vi "BatteryWarningTest_3.6V.vi"(8 "error in":errorcluster) -> (0 "error in (no error)":errorcluster, 1 "Pass/Fail":bool, 4 "Limit2":u8[](array[numeric]) format="%x", 5 "Limit1":u8[](array[numeric]) format="%x")   [LabVIEW 2009]
uses:
  Global/Global 1.vi
  <vilib>/Instr/_visa.llb/VISA Configure Serial Port (Instr).vi
panel:
  # "30"
  # "0A"
  # "30"
  # "0A"
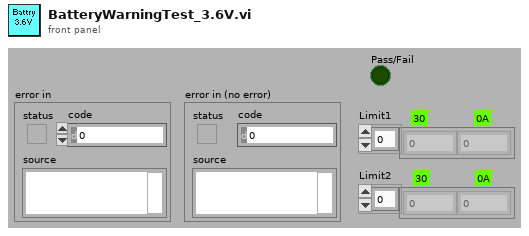
[diagram p1: front panel]
types:
  T1 = cluster{"VHEATFUSENOLOADMIN":string, "VHEATFUSELOADMAX":string, "VOVERRIDEDIODEMIN":string, "TDIFFMAX":string, "MEASFREQMAX":string, "MEASFREQMIN":string, "VOVER":string, "VMIDDLE":string, "VUNDER":string, "VNORESET":string, "VRESET":string, "WAITPING":string, "LRFID":string, "RFIDUID":string, "EXTEESIZE":string, "LCUTYPE":string, "LCUSUBTYPE":string, "TEVN":string, "BOOTVER":string, "APPVER":string, "ISLEEPMAX":string, "TSLEEP":string, "APPWAIT":string, "DBWAIT":string}
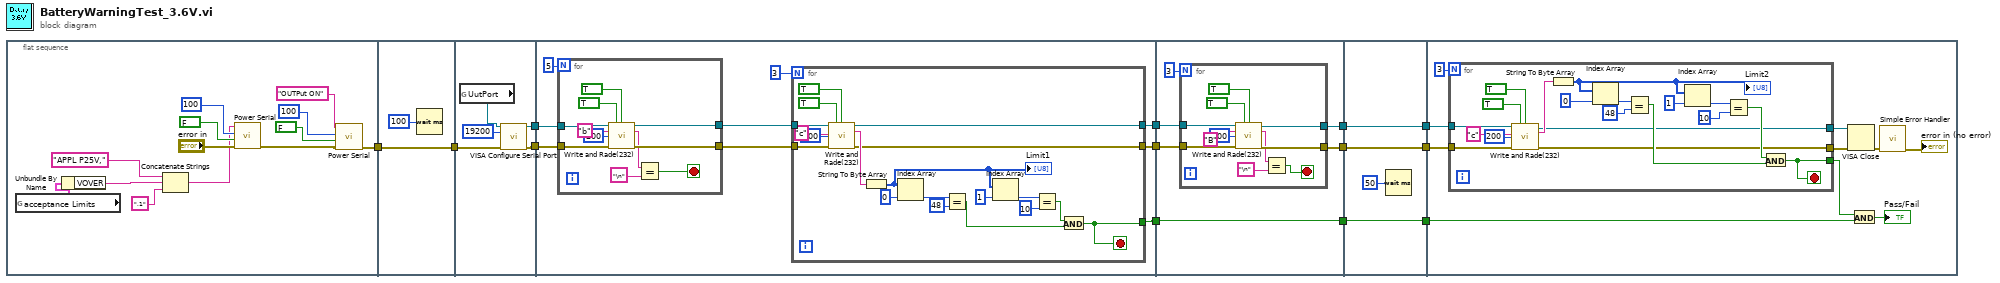
[diagram p0: block diagram]
diagram:
  n1 = flat-sequence {
    tunnel: [w19] -> w2
    tunnel: w2 -> [w28]
    tunnel: [w28] -> w1
    tunnel: [w33] -> w5
    tunnel: [w32] -> w4
    tunnel: w1 -> [w30]
    tunnel: [w42] -> w11
    tunnel: [w41] -> w6
    tunnel: [w38] -> w3
    tunnel: w4 -> [w35]
    tunnel: w5 -> [w36]
    tunnel: [w78] -> w12
    tunnel: w11 -> [w78]
    tunnel: [w77] -> w10
    tunnel: [w76] -> w8
    tunnel: w6 -> [w75]
    tunnel: w3 -> [w74]
    tunnel: [w92] -> w13
    tunnel: w12 -> [w92]
    tunnel: w10 -> [w91]
    tunnel: [w91] -> w9
    tunnel: w8 -> [w90]
    tunnel: [w90] -> w7
    tunnel: w13 -> [w102]
    tunnel: w9 -> [w100]
    tunnel: w7 -> [w99]
    frame #0 {
      n2 = global read "Global 1.vi" "acceptance Limits"() -> (w18:T1)
      n3 = Unbundle By Name(w18) -> ("VOVER"=w17:string)
      n4 = Concatenate Strings("APPL P25V," ("In"), w17, ",1" ("string")) -> (w14:string)
      n5 = call "Power Serial.vi"("error in (no error)"="error in", "Rd?"=FALSE, "Delay"=100, "IN"=w14) -> ("error out"=w23:errorcluster)  [unwired: 1 in, 6 out]
      n6 = call "Power Serial.vi"("error in (no error)"=w23, "Rd?"=FALSE, "Delay"=100, "IN"="OUTPut ON" ("In")) -> ("error out"=w19:errorcluster)  [unwired: 1 in, 6 out]
    }
    frame #1 {
      n7 = Wait (ms)(milliseconds to wait=u32 100) -> ()  [unwired: 1 out]
    }
    frame #2 {
      n8 = global read "Global 1.vi" "UutPort"() -> (w29:refnum<visa-resource-name>)
      n9 = call-poly "VISA Configure Serial Port"("VISA resource name"=w29, "baud rate (9600)"=u32 19200, "error in (no error)"=w30) -> ("VISA resource name out"=w32:refnum<visa-resource-name>, "error out"=w33:errorcluster)  [unwired: 3 in, 8 out]
    }
    frame #3 {
      n10 = for {
        N: 5 -> [_]
        tunnel: [w50] -> w40
        tunnel: w36 -> [w49]
        tunnel: w35 -> [w48]
        tunnel: [w47] -> w39
        stop <- w44 stop-if-true
        n11 = call "Write and Rade(232).vi"("VISA resource name in"=w48, "write"=TRUE, "read"=TRUE, "string to write"="b", "ms delay"=u32 200, "error in"=w49) -> ("VISA resource name out"=w50:refnum<visa-resource-name>, "read string"=w46:string, "error out"=w47:errorcluster)  [unwired: 2 in, 5 out]
        n12 = Equal?(x=w46, y="\n") -> (x = y?=w44:bool)
      }
      n13 = for {
        N: 3 -> [_]
        tunnel: [w55] -> w42
        tunnel: [w59] -> w41
        tunnel: w40 -> [w58]
        tunnel: w39 -> [w57]
        tunnel: [w56] -> w38
        stop <- w55 stop-if-true
        n14 = call "Write and Rade(232).vi"("VISA resource name in"=w58, "write"=TRUE, "read"=TRUE, "string to write"="c", "ms delay"=u32 200, "error in"=w57) -> ("VISA resource name out"=w59:refnum<visa-resource-name>, "read string"=w61:string, "error out"=w56:errorcluster)  [unwired: 2 in, 5 out]
        n15 = String To Byte Array(string=w61) -> (unsigned byte array=w67:u8[])
        "Limit1" <- w67
        n16 = Index Array(array=w67, index=0) -> (element=w65:u8)
        n17 = Equal?(x=w65, y=u8 48) -> (x = y?=w72:bool)
        n18 = Index Array(array=w67, index=1) -> (element=w69:u8)
        n19 = Equal?(x=w69, y=u8 10) -> (x = y?=w71:bool)
        n20 = And(x=w71, y=w72) -> (x .and. y?=w55:bool)
      }
    }
    frame #4 {
      n21 = for {
        N: 3 -> [_]
        tunnel: [w86] -> w77
        tunnel: [w85] -> w76
        tunnel: w75 -> [w84]
        tunnel: w74 -> [w83]
        stop <- w80 stop-if-true
        n22 = call "Write and Rade(232).vi"("VISA resource name in"=w84, "write"=TRUE, "read"=TRUE, "string to write"="B", "ms delay"=u32 200, "error in"=w83) -> ("VISA resource name out"=w85:refnum<visa-resource-name>, "read string"=w82:string, "error out"=w86:errorcluster)  [unwired: 2 in, 5 out]
        n23 = Equal?(x=w82, y="\n") -> (x = y?=w80:bool)
      }
    }
    frame #5 {
      n24 = Wait (ms)(milliseconds to wait=u32 50) -> ()  [unwired: 1 out]
    }
    frame #6 {
      n25 = for {
        N: 3 -> [_]
        tunnel: [w105] -> w103
        tunnel: w100 -> [w110]
        tunnel: w99 -> [w108]
        tunnel: [w107] -> w96
        tunnel: [w106] -> w95
        stop <- w105 stop-if-true
        n26 = call "Write and Rade(232).vi"("VISA resource name in"=w108, "write"=TRUE, "read"=TRUE, "string to write"="c", "ms delay"=u32 200, "error in"=w110) -> ("VISA resource name out"=w106:refnum<visa-resource-name>, "read string"=w109:string, "error out"=w107:errorcluster)  [unwired: 2 in, 5 out]
        n27 = String To Byte Array(string=w109) -> (unsigned byte array=w118:u8[])
        "Limit2" <- w118
        n28 = Index Array(array=w118, index=0) -> (element=w116:u8)
        n29 = Equal?(x=w116, y=u8 48) -> (x = y?=w122:bool)
        n30 = Index Array(array=w118, index=1) -> (element=w120:u8)
        n31 = Equal?(x=w120, y=u8 10) -> (x = y?=w114:bool)
        n32 = And(x=w114, y=w122) -> (x .and. y?=w105:bool)
      }
      n33 = VISA Close(VISA resource name=w95, error in (no error)=w96) -> (error out=w97:errorcluster)
      n34 = And(x=w103, y=w102) -> (x .and. y?=→"Pass/Fail":bool)
      n35 = call <vilib>:"Simple Error Handler.vi"("error in (no error)"=w97) -> ("error out"=→"error in (no error)":errorcluster)  [unwired: 1 in, 7 out]
    }
  }
